vi "_skipWhiteSpace.vi"(8 "error in (no error)":errorcluster, 11 "JSON Parser In":refnum<class "tJSONParser.lvclass">=refnum) -> (0 "error out":errorcluster, 1 "EOL Found?":bool, 2 "White Space Found?":bool, 3 "JSON Parser Out":refnum<class "tJSONParser.lvclass">, 5 "Whitespace String":string)   [LabVIEW 2013, in "JSON.lvlib" / "tJSONParser.lvclass"]
doc: "Removes all leading white space from a JSON string. Also increments the line number when an EOL is found. The whitespace string that was found is returned as 'Whitespace String'."
uses:
  tJSONParser.lvclass
  tJSONParser.lvclass/tJSONParser.ctl
  <vilib>/regexp/Match Regular Expression.xnode
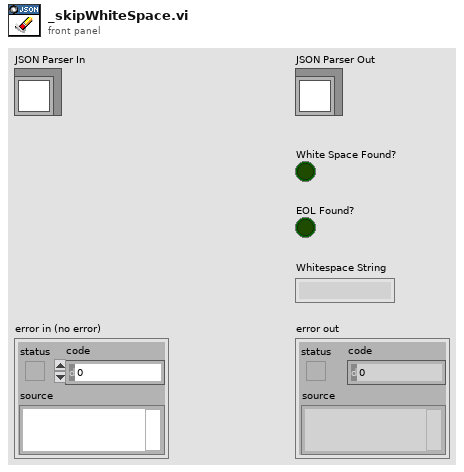
[diagram p1: front panel]
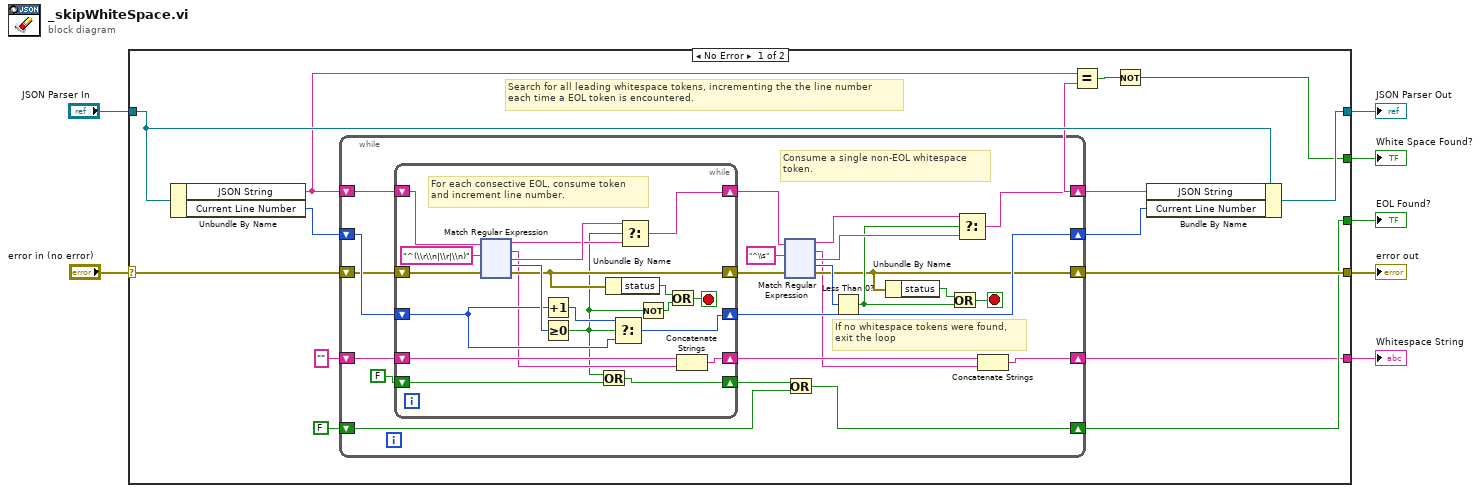
[diagram p0: block diagram]
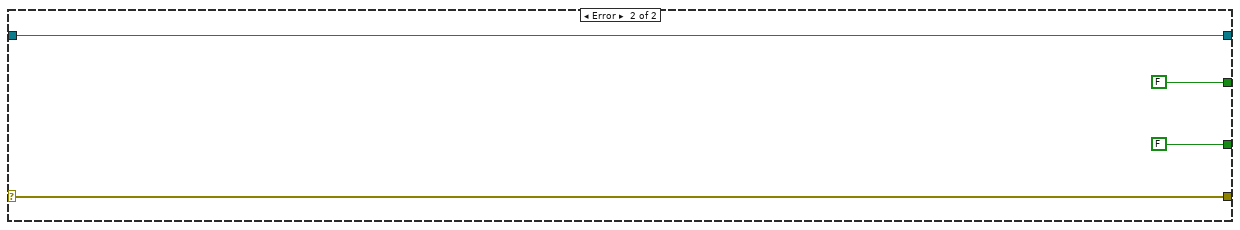
[diagram p2: hidden frame]
diagram:
  n1 = case shown="No Error" "error in (no error)" {
    selector: "error in (no error)" -> [w21 w290]
    tunnel: [w20 w290] -> w6
    tunnel: "JSON Parser In" -> [w19 w289]
    tunnel: [w18 w289] -> w5
    tunnel: [w8 FALSE] -> w3
    tunnel: [w15 FALSE] -> w2
    tunnel: [w12 _] -> w1
    frame No Error {
      # "Search for all leading whitespace tokens, incrementing the the line number\neach time a EOL token is encountered."
      n2 = Unbundle By Name(w19) -> ("JSON String"=w11:string, "Current Line Number"=w17:u32)
      n3 = while {
        shift-right: [w36] -> w10
        shift-left: w11 -> [w40]
        shift-right: [w37] -> w16
        shift-left: w17 -> [w39]
        shift-right: [w30] -> w20
        shift-left: w21 -> [w38]
        shift-right: [w27] -> w15
        shift-left: FALSE -> [w28]
        shift-right: [w25] -> w12
        shift-left: "" -> [w26]
        stop <- w33 stop-if-true
        # "If no whitespace tokens were found,\nexit the loop"
        # "Consume a single non-EOL whitespace\ntoken."
        n4 = while {
          shift-right: [w170] -> w37
          shift-left: w39 -> [w169]
          shift-right: [w164] -> w44
          shift-left: w40 -> [w173]
          shift-right: [w168] -> w43
          shift-left: w38 -> [w175]
          shift-right: [w161] -> w24
          shift-left: w26 -> [w160]
          shift-right: [w157] -> w29
          shift-left: FALSE -> [w158]
          stop <- w165 stop-if-true
          # "For each consective EOL, consume token\nand increment line number."
          n5 = xnode "Match Regular Expression"("input string"=w173, "regular expression"="^(\\r\\n|\\r|\\n)", "error in"=w175) -> ("before match"=w162:string, "whole match"=w159:string, "after match"=w163:string, "offset past match"=w172:i32, "error out"=w168:errorcluster)  [unwired: 3 in]
          n6 = Increment(x=w169) -> (x+1=w171:u32)
          n7 = Greater Or Equal To 0?(x=w172) -> (x >= 0?=w156:bool)
          n8 = Or(x=w156, y=w158) -> (x .or. y?=w157:bool)
          n9 = Unbundle By Name(w168) -> ("status"=w166:bool)
          n10 = Select(t=w171, s=w156, f=w169) -> (s? t:f=w170:u32)
          n11 = Select(t=w163, s=w156, f=w162) -> (s? t:f=w164:string)
          n12 = Not(x=w156) -> (.not. x?=w167:bool)
          n13 = Or(x=w166, y=w167) -> (x .or. y?=w165:bool)
          n14 = Concatenate Strings(w160, w159) -> (w161:string)
        }
        n15 = xnode "Match Regular Expression"("input string"=w44, "regular expression"="^\\s", "error in"=w43) -> ("before match"=w35:string, "whole match"=w23:string, "after match"=w34:string, "offset past match"=w41:i32, "error out"=w30:errorcluster)  [unwired: 3 in]
        n16 = Or(x=w29, y=w28) -> (x .or. y?=w27:bool)
        n17 = Less Than 0?(x=w41) -> (x < 0?=w31:bool)
        n18 = Unbundle By Name(w30) -> ("status"=w32:bool)
        n19 = Or(x=w32, y=w31) -> (x .or. y?=w33:bool)
        n20 = Select(t=w35, s=w31, f=w34) -> (s? t:f=w36:string)
        n21 = Concatenate Strings(w24, w23) -> (w25:string)
      }
      n22 = Equal?(x=w11, y=w10) -> (x = y?=w9:bool)
      n23 = Not(x=w9) -> (.not. x?=w8:bool)
      n24 = Bundle By Name(cluster=w19, "JSON String"=w10, "Current Line Number"=w16) -> (w18:refnum<class "tJSONParser.lvclass">)
    }
    frame Error {
    }
  }
  "error out" <- w6
  "JSON Parser Out" <- w5
  "White Space Found?" <- w3
  "EOL Found?" <- w2
  "Whitespace String" <- w1
